vi "Main.vi"() -> ()   [LabVIEW 2022 SP3]
uses:
  <vilib>/Platform/TimedLoop/XDataNode/timing_clust.ctl
  <vilib>/Platform/TimedLoop/XDataNode/nitl_modes.ctl
  <vilib>/Platform/TimedLoop/XDataNode/wakeup.ctl
  <vilib>/platform/TimedLoop/XDataNode/XDataNode.xnode
  <vilib>/Platform/TimedLoop/XDataNode/XDNodeRunTimeDep.lvlib
panel:
  out "waypoints":dbl[][](array[numeric])
  out "waypointsSize":i32
  out "indicator":dbl
  out "bruh":dbl[][](array[numeric])
  out "cuuurrentpad":dbl[][](array[numeric])
  out "angle":dbl
  out "XY Graph 2":cluster{dbl[], dbl[]}[](graph)
  in  "Straal":dbl=5.0
  in  "Filter on/off":bool
  in  "Speed":dbl=3.0
  out "XY Graph":cluster{dbl[], dbl[]}[](graph)
  in  "stop":bool
  in  "Aantal hoekken":dbl=5.0
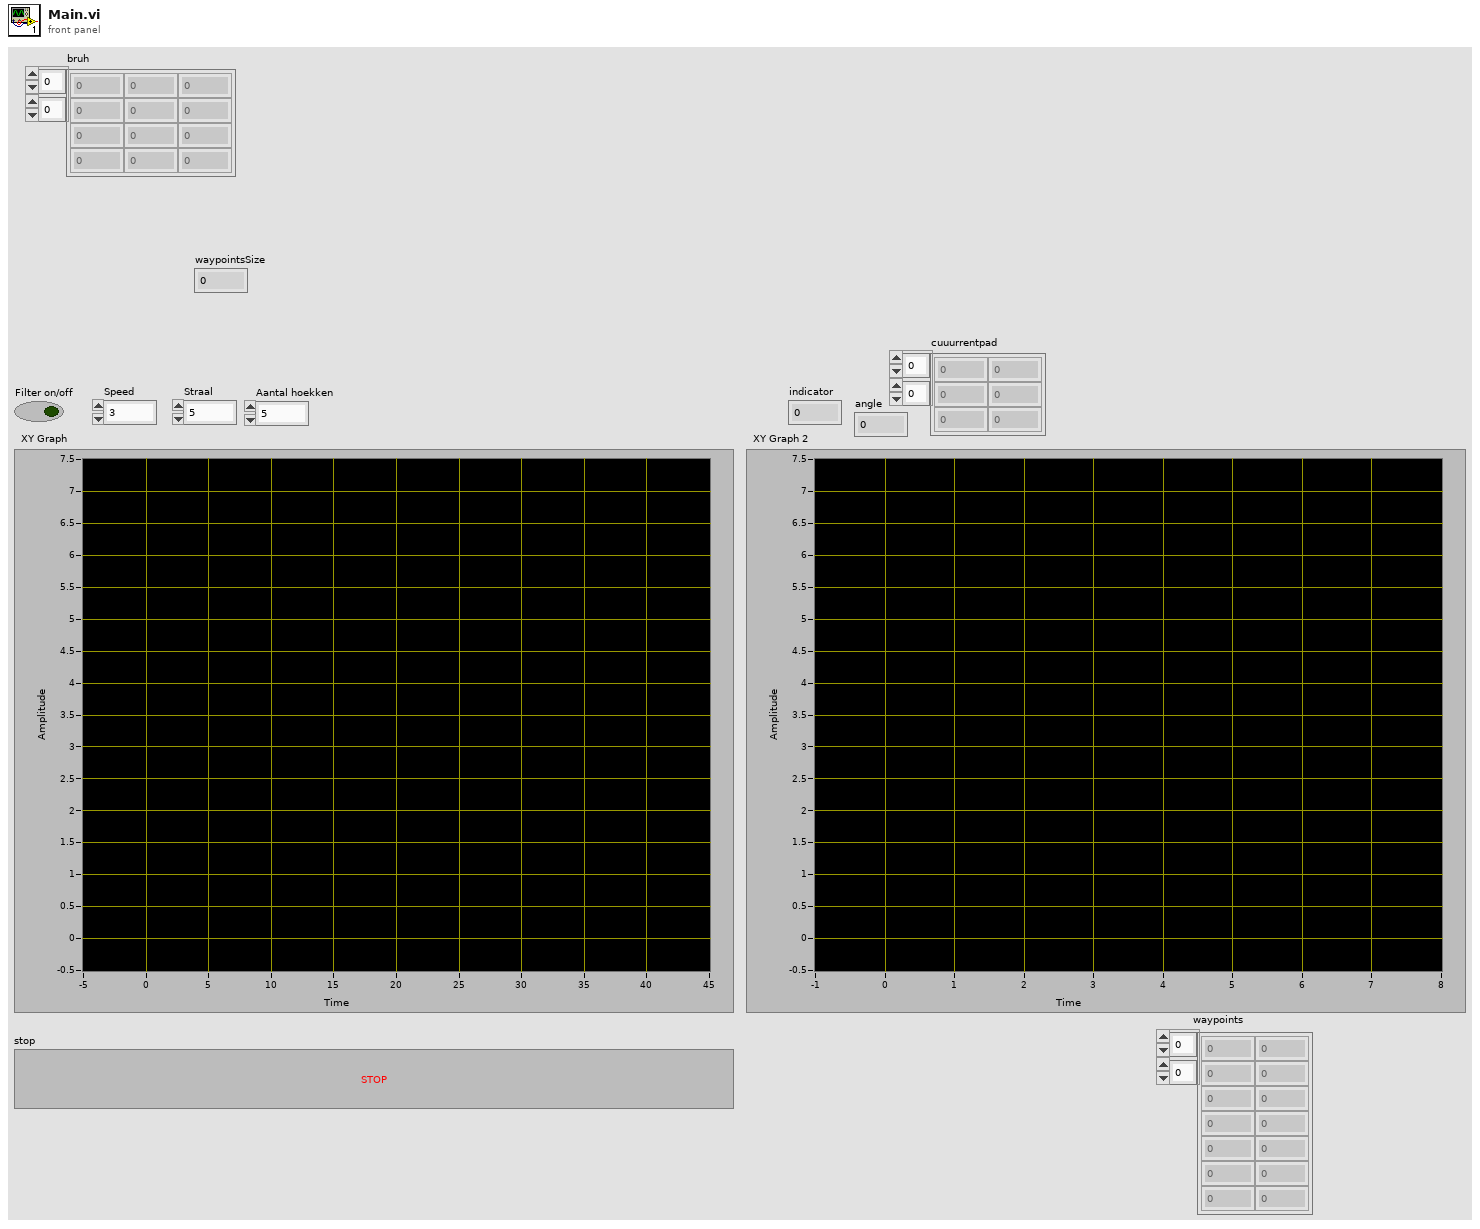
[diagram p1: front panel]
types:
  T1 = typedef "XDNodeRunTimeDep.lvlib/timing_clust.ctl" = cluster{"Expected End [f-1]":u64, "Actual End [f-1]":u64, "Finished Late? [f-1]":bool, "Expected End [i-1]":u64, "Actual End [i-1]":u64, "Finished Late? [i-1]":bool, "Expected Start [i]":u64, "Actual Start [i]":u64, "Expected Start [f]":u64, "Actual Start [f]":u64, "Source Name":string, "Structure Name":string, "Period":i64, "Deadline":i64, "Offset":i64, "Start":i64, "Priority":i32, "Timeout":i32, "Mode":T2, "Wakeup Reason":T3, "Error":errorcluster, "Source Type":string, "Secondary Source Type":string, "Global End Time":u64, "Global Start Time":u64, "Frame Duration":u64, "Iteration Duration":u64, "Assigned CPU":i32, "I/O Scan Engine Mode":u32}
  T2 = typedef "XDNodeRunTimeDep.lvlib/nitl_modes.ctl" = enum32{"No Change", "Process missed periods, maintain original phase", "Discard missed periods, maintain original phase", "Process missed periods, ignore original phase", "Discard missed periods, ignore original phase"}
  T3 = typedef "XDNodeRunTimeDep.lvlib/wakeup.ctl" = enum32{"Normal", "Aborted", "Asynchronous wakeup", "Timing source error", "Timed loop error", "Timeout"}
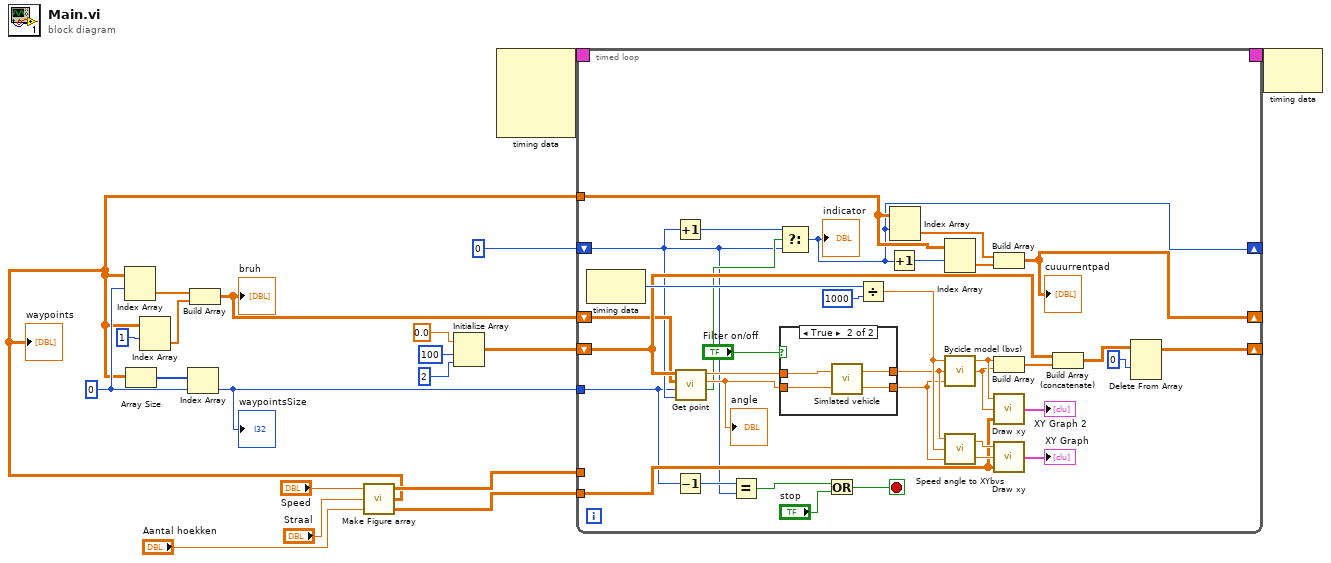
[diagram p0: block diagram]
diagram:
  w3 = 0
  n1 = call "Make Figure array.vi"("Aantal hoekken (n)"="Aantal hoekken", "Straal (s)"="Straal", "Speed"="Speed") -> ("Figur array"=w14:dbl[][], "waypoints"=w1:dbl[][], "Route Array"=w15:dbl[][])
  "waypoints" <- w1
  n2 = Index Array(array=w1, index (row)=w3) -> (element=w7:dbl[])  [unwired: 1 in]
  n3 = Array Size(array=w1) -> (size(s)=w4:i32[])
  n4 = Index Array(array=w1, index (row)=1) -> (element=w6:dbl[])  [unwired: 1 in]
  n5 = Index Array(array=w4, index=w3) -> (element=w2:i32)
  "waypointsSize" <- w2
  n6 = Build Array(w7, w6) -> (w8:dbl[][])
  "bruh" <- w8
  n7 = Initialize Array(0.0, 100, 2) -> (w10:dbl[][])
  n8 = node-c288() -> (w20:T1)  [unwired: 4 in]
  n9 = timed-loop {
    timing: w20 -> [_]
    timing-out: [_] -> w19
    tunnel: w15 -> [_]
    tunnel: w14 -> [w42]
    shift-right: [w40] -> _
    shift-left: w10 -> [w37]
    tunnel: w1 -> [w30]
    shift-right: [w27] -> _
    shift-left: w8 -> [w26]
    shift-right: [w25] -> _
    shift-left: 0 -> [w23]
    tunnel: w2 -> [w21]
    stop <- w54 stop-if-true
    n10 = node-c288() -> (w53:i64)  [unwired: 1 in]
    n11 = Increment(x=w23) -> (x+1=w33:i32)
    n12 = Decrement(x=w21) -> (x-1=w24:i32)
    n13 = call "Get point.vi"("current index"=w23, "lenghtWaypointList"=w21, "currentPath"=w26, "posList"=w37) -> ("check"=w32:bool, "Angle"=w35:dbl, "Speed"=w50:dbl)  [unwired: 1 out]
    "angle" <- w35
    n14 = Equal?(x=w24, y=w23) -> (x = y?=w22:bool)
    n15 = Select(t=w33, s=w32, f=w23) -> (s? t:f=w25:i32)
    "indicator" <- w25
    n16 = case shown="True" "Filter on/off" {
      tunnel: w50 -> [w57 w61]
      tunnel: [w57 w60] -> w45
      tunnel: [w56 w59] -> w44
      tunnel: w35 -> [w56 w58]
      frame False {
      }
      frame True {
        n17 = call "Simlated vehicle.vi"("Steering angle"=w58, "Speed"=w61) -> ("Steering angle sensor"=w59:dbl, "Speed sensor"=w60:dbl)
      }
    }
    n18 = Or(x=w22, y="stop") -> (x .or. y?=w54:bool)
    n19 = Divide(x=w53, y=i64 1000) -> (x/y=w46:dbl)
    n20 = Increment(x=w25) -> (x+1=w31:i32)
    n21 = Index Array(array=w30, index (row)=w25) -> (element=w28:dbl[])  [unwired: 1 in]
    n22 = Index Array(array=w30, index (row)=w31) -> (element=w29:dbl[])  [unwired: 1 in]
    n23 = call "Bycicle model (bvs).vi"("Wheel angle (deg)"=w44, "Ground speed (km/h)"=w45, "dt (s)"=w46) -> ("New position Y"=w38:dbl, "New position X"=w39:dbl)  [unwired: 1 out]
    n24 = call "Speed angle to XYbvs.vi"("Angle(deg)"=w44, "dt(s)"=w46, "Speed(km/h)"=w45) -> ("Y"=w47:dbl, "x"=w48:dbl)
    n25 = Build Array(w28, w29) -> (w27:dbl[][])
    "cuuurrentpad" <- w27
    n26 = Build Array(w39, w38) -> (w34:dbl[])
    n27 = call "Draw xy.vi"("Figur array"=w42, "Y"=w38, "x"=w39) -> ("XY Graph"=→"XY Graph 2":cluster{dbl[], dbl[]}[])
    n28 = call "Draw xy.vi"("Figur array"=w42, "Y"=w47, "x"=w48) -> ("XY Graph"=→"XY Graph":cluster{dbl[], dbl[]}[])
    n29 = Build Array (concatenate)(w37, w34) -> (w41:dbl[][])
    n30 = Delete From Array(array=w41, index (row)=0) -> (array with subset deleted=w40:dbl[][])  [unwired: 2 in, 1 out]
  }
  n31 = node-c288(w19) -> ()  [unwired: 1 out]
